vi "Dual Digital Oscilliscope%255bExpress%255d.vi"() -> ()   [LabVIEW 2015]
panel:
  out "error out":errorcluster
  out "source":string
  in  "Digitizing Parameters":T1
  out "Waveform Graph":dynamicdata(graph)
  in  "stop":bool
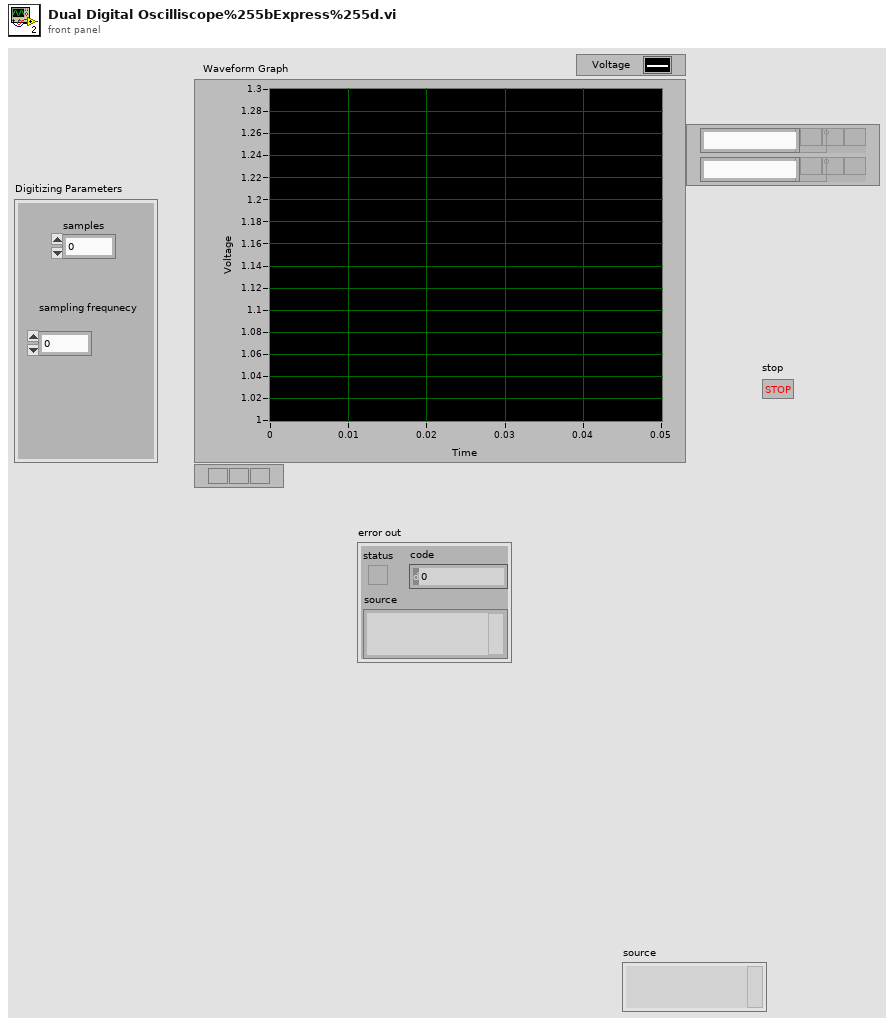
[diagram p1: front panel]
types:
  T1 = cluster{"samples":dbl, "sampling frequnecy\n":dbl}
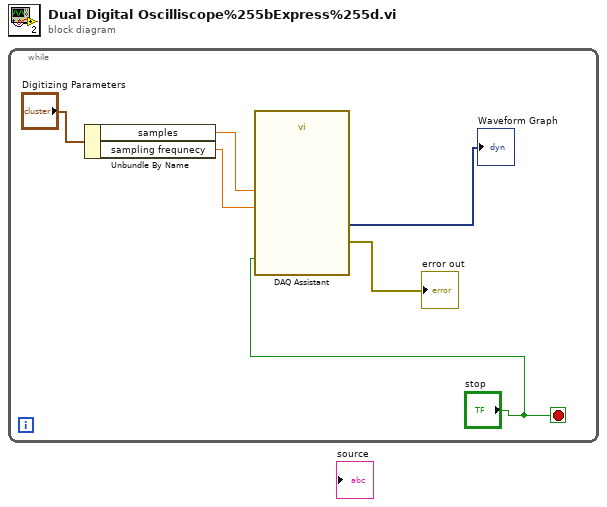
[diagram p0: block diagram]
diagram:
  n1 = while {
    stop <- "stop" stop-if-true
    n2 = Unbundle By Name("Digitizing Parameters") -> ("samples"=w3:dbl, "sampling frequnecy"=w2:dbl)
    n3 = call "DAQ Assistant"("rate"=w2, "number of samples"=w3, "stop (T)"="stop") -> ("data"=→"Waveform Graph":dynamicdata, "error out"=→"error out":errorcluster)  [unwired: 14 in, 1 out]
  }
